vi "Write configuration.vi"(8 "error in":errorcluster, 10 "configuration":refnum<class "NISE_CEF_serializable configuration.lvclass">, 11 "PLTarget PC in":refnum<class "PLTarget PC.lvclass">) -> (0 "error out":errorcluster, 3 "PLTarget PC out":refnum<class "PLTarget PC.lvclass">)   [LabVIEW 2013, in "PLTarget PC.lvclass"]
uses:
  PLTarget PC.lvclass
  Framework Configuration Classes/target configuration/PL_Target Configuration.lvclass
  <vilib>/NI/CEF/CEF_TreeControl/serializable configuration/NISE_CEF_serializable configuration.lvclass
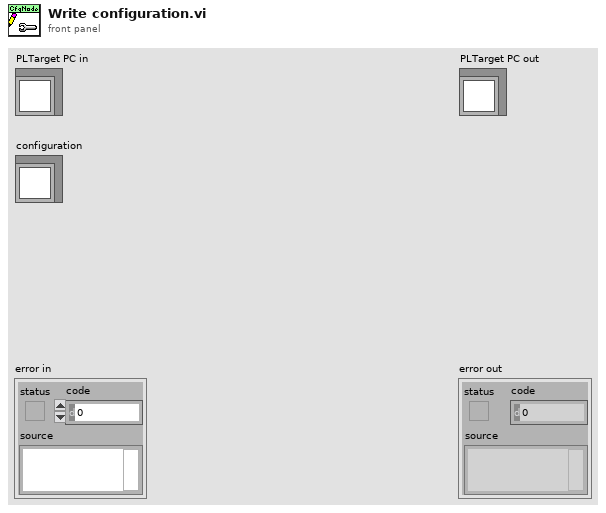
[diagram p1: front panel]
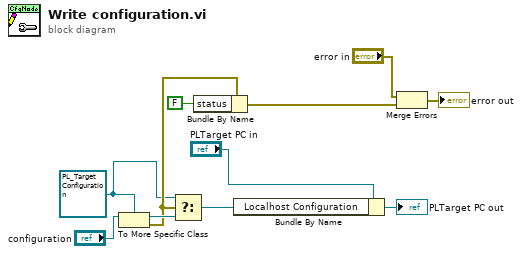
[diagram p0: block diagram]
diagram:
  w7 = refnum<class "PL_Target Configuration.lvclass"> refnum ("Local Target Configuration")
  n1 = To More Specific Class(target class=w7, reference="configuration") -> (specific class reference=w11:refnum<class "PL_Target Configuration.lvclass">, error out=w10:errorcluster)  [unwired: 1 in]
  n2 = Select(t=w7, s=w10, f=w11) -> (s? t:f=w6:refnum<class "PL_Target Configuration.lvclass">)
  n3 = Bundle By Name(cluster=w10, "status"=FALSE) -> (w8:errorcluster)
  n4 = Bundle By Name(cluster="PLTarget PC in", "Localhost Configuration"=w6) -> (→"PLTarget PC out":refnum<class "PLTarget PC.lvclass">)
  n5 = Merge Errors("error in", w8) -> (→"error out":errorcluster)
